vi "support_locateDataDir.vi"(8 "error in (no error)":errorcluster) -> (0 "error out":errorcluster, 3 "data folder Dir":path)   [LabVIEW 2010]
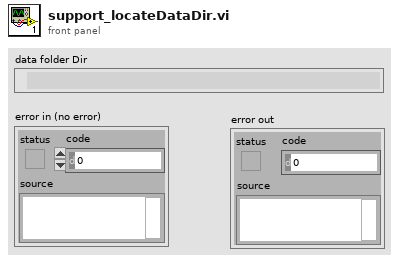
[diagram p1: front panel]
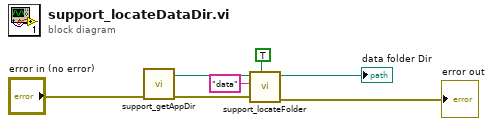
[diagram p0: block diagram]
diagram:
  n1 = call "support_getAppDir.vi"("error in (no error)"="error in (no error)") -> ("error out"=w5:errorcluster, "App.Dir"=w6:path)  [unwired: 9 in]
  n2 = call "support_locateFolder.vi"("create if not found?"=TRUE, "error in (no error)"=w5, "Folder"="data" ("folder"), "Root"=w6) -> ("error IO"=→"error out":errorcluster, "path"=→"data folder Dir":path)  [unwired: 5 in, 1 out]
